vi "Disconnect OPC UA.vi"(8 "error in (no error)":errorcluster, 11 "FGV Name":string="PLC Ref") -> (0 "error out":errorcluster)   [LabVIEW 2021, in "OPC UA.lvlib" / "OPC UA.lvclass"]
uses:
  OPC UA.lvclass
  <vilib>/OPCUA/controls/OPC UA Client Refnum.ctl
  OPC UA.lvclass/OPC UA.ctl
  <vilib>/OPCUA/NI OPC UA Client.lvlib
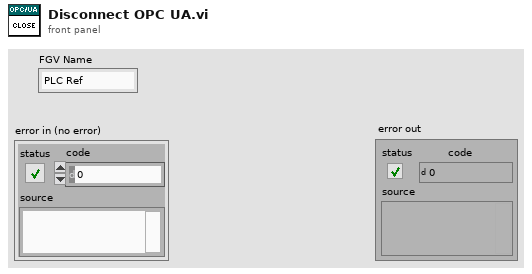
[diagram p1: front panel]
types:
  T1 = typedef "OPC UA Client Refnum.ctl" = refnum<k21>
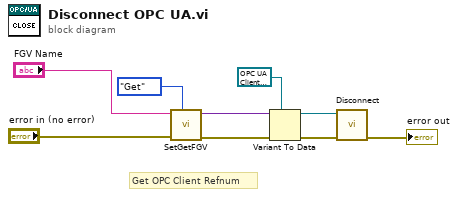
[diagram p0: block diagram]
diagram:
  # "Get OPC Client Refnum"
  n1 = call "SetGetFGV.vi"("Method (Get)"=enum16{"Get", "Set"}."Get", "error in"="error in (no error)", "Name"="FGV Name") -> ("error out"=w4:errorcluster, "Data out"=w3:variant)  [unwired: 7 in]
  n2 = Variant To Data(error in=w4, type=T1 refnum ("OPC UA client refnum out"), Variant=w3) -> (data=w7:T1, error out=w6:errorcluster)
  n3 = call <vilib>:"Disconnect.vi"("error in (no error)"=w6, "OPC UA client refnum in"=w7) -> ("error out"=→"error out":errorcluster)  [unwired: 9 in]
